vi "nchans.vi"(1 "channels":string) -> (0 "length (rest)":i32)   [LabVIEW 2010]
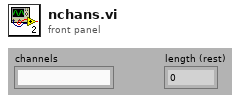
[diagram p1: front panel]
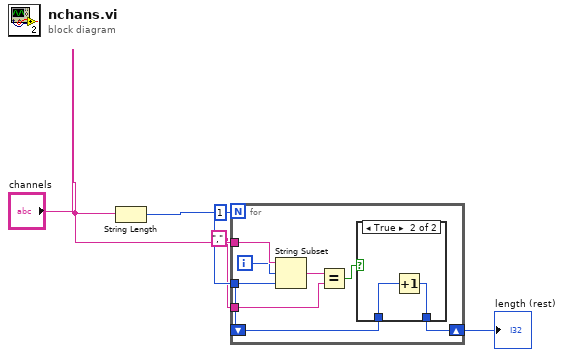
[diagram p0: block diagram]
diagram:
  w2 = 1 ("length (rest)")
  n1 = String Length(string="channels") -> (length=w5:i32)
  n2 = for {
    N: w5 -> [_]
    tunnel: "channels" -> [w13]
    tunnel: w2 -> [w11]
    tunnel: "," ("y") -> [w9]
    shift-right: [w7] -> w3
    shift-left: w2 -> [w6]
    i -> [w12]
    n3 = String Subset(string=w13, offset (0)=w12, length (rest)=w11) -> (substring=w10:string)
    n4 = Equal?(x=w10, y=w9) -> (x = y?=w8:bool)
    n5 = case shown="True" w8 {
      tunnel: [w14 w16] -> w7
      tunnel: w6 -> [w14 w15]
      frame False {
      }
      frame True {
        n6 = Increment(x=w15) -> (x+1=w16:i32)
      }
    }
  }
  "length (rest)" <- w3
